vi "LJstreamUD get file name.vi"(9 "Starting #":u32, 10 "Data File Prefix":string="data", 11 "Working Directory":path) -> (1 "Data File #":u32, 3 "Data File Path":path)   [LabVIEW 2020]
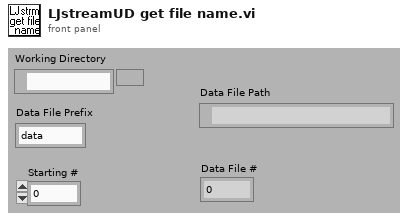
[diagram p1: front panel]
types:
  T1 = enum16{"open", "replace", "create", "open or create", "replace or create", "replace or create with confirmation"}
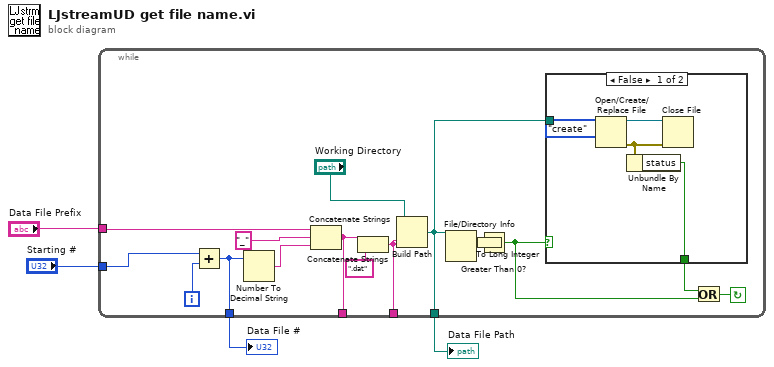
[diagram p0: block diagram]
diagram:
  n1 = while {
    tunnel: [w6] -> w1
    tunnel: "Starting #" -> [w8]
    tunnel: [w14] -> _
    tunnel: [w13] -> w3
    tunnel: [w16] -> _
    tunnel: "Data File Prefix" -> [w18]
    i -> [w7]
    stop <- w12 continue-if-true
    n2 = Add(x=w8, y=w7) -> (x+y=w6:u32)
    n3 = Number To Decimal String(number=w6) -> (decimal integer string=w20:string)  [unwired: 1 in]
    n4 = Concatenate Strings(w18, "_" ("Substring"), w20) -> (w14:string)
    n5 = Concatenate Strings(w14, ".dat" ("Substring")) -> (w16:string)
    n6 = Build Path(base path="Working Directory", name or relative path=w16) -> (appended path=w13:path)
    n7 = File/Directory Info(path=w13) -> (size=w5:i64)  [unwired: 1 in, 6 out]
    n8 = To Long Integer(number=w5) -> (32bit integer=w19:i32)
    n9 = Greater Than 0?(x=w19) -> (x > 0?=w9:bool)
    n10 = case shown="False" w9 {
      selector: w9 -> [_ w26]
      tunnel: w13 -> [w25 _]
      tunnel: [w23 w26] -> w11
      frame False {
        n11 = Open/Create/Replace File(file path (use dialog)=w25, operation (0:open)=T1."create") -> (refnum out=w22:refnum<file>, error out=w24:errorcluster)  [unwired: 4 in, 1 out]
        n12 = Unbundle By Name(w24) -> ("status"=w23:bool)
        n13 = Close File(refnum=w22, error in=w24) -> ()  [unwired: 2 out]
      }
      frame True {
      }
    }
    n14 = Or(x=w11, y=w9) -> (x .or. y?=w12:bool)
  }
  "Data File Path" <- w3
  "Data File #" <- w1
